vi "Subvi Acquire Multiple Image.vi"(2 "ImageRepeatNum":u32, 3 "InFileName":string) -> (0 "ImgAbort":bool, 1 "ImgTaken":bool)   [LabVIEW 2012]
panel:
  out "FinalFileName":string
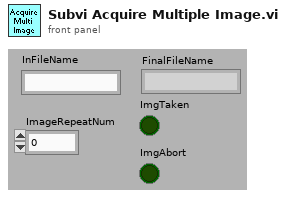
[diagram p1: front panel]
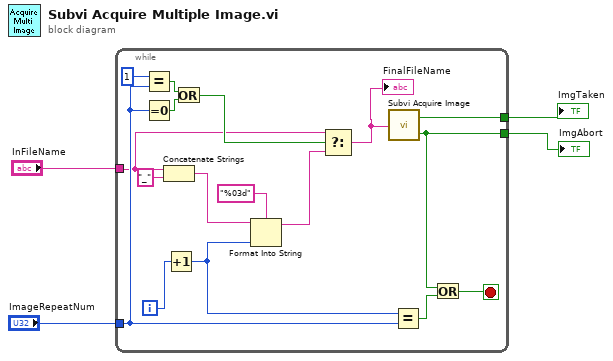
[diagram p0: block diagram]
diagram:
  n1 = while {
    tunnel: "InFileName" -> [w7]
    tunnel: "ImageRepeatNum" -> [w11]
    tunnel: [w14] -> w4
    tunnel: [w13] -> w3
    i -> [w21]
    stop <- w18 stop-if-true
    n2 = Equal?(x=u32 1, y=w11) -> (x = y?=w12:bool)
    n3 = Equal To 0?(x=w11) -> (x = 0?=w10:bool)
    n4 = Concatenate Strings(w7, "_" ("string")) -> (w15:string)
    n5 = Increment(x=w21) -> (x+1=w16:i32)
    n6 = Or(x=w12, y=w10) -> (x .or. y?=w8:bool)
    n7 = Format Into String(format string="%03d", initial string=w15, w16) -> (resulting string=w6:string)  [unwired: 1 in, 1 out]
    n8 = Select(t=w7, s=w8, f=w6) -> (s? t:f=w5:string)
    "FinalFileName" <- w5
    n9 = call "Subvi Acquire Image.vi"("ImgFile"=w5) -> ("ImgTaken"=w14:bool, "ImgAbort"=w13:bool)
    n10 = Equal?(x=w16, y=w11) -> (x = y?=w19:bool)
    n11 = Or(x=w13, y=w19) -> (x .or. y?=w18:bool)
  }
  "ImgTaken" <- w4
  "ImgAbort" <- w3
